vi "RT Loop - Log Data.vi"(8 "error in (no error)":errorcluster, 9 "Acceleration RT FIFO In":T1, 11 "Message Queue":refnum<queue>) -> ()   [LabVIEW 2017]
doc: "Receive triggered data from Analyze Acceleration Loop and log the data to disk."
uses:
  C:/Users/me1hlx/Desktop/Embedded Control and Monitoring/Exercises/Sample Project/support/Message Queue/Message Cluster.ctl
  C:/Users/me1hlx/Desktop/Embedded Control and Monitoring/Exercises/Sample Project/controls/Acceleration RT FIFO Reference.ctl
  C:/Users/me1hlx/Desktop/Embedded Control and Monitoring/Exercises/Sample Project/Globals/Global - All RT Loop Stop.vi
  C:/Users/me1hlx/Desktop/Embedded Control and Monitoring/Exercises/Sample Project/Globals/Global - Configuration Options.vi
  C:/Users/me1hlx/Desktop/Embedded Control and Monitoring/Exercises/Sample Project/support/Logging/Logging.lvlib
  C:/Users/me1hlx/Desktop/Embedded Control and Monitoring/Exercises/Sample Project/support/Message Queue/Message Queue.lvlib
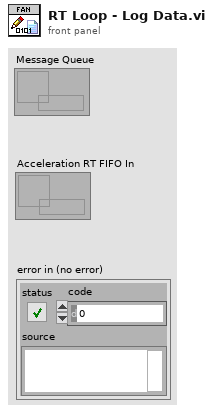
[diagram p1: front panel]
types:
  T1 = typedef "Acceleration RT FIFO Reference.ctl" = refnum<k33>
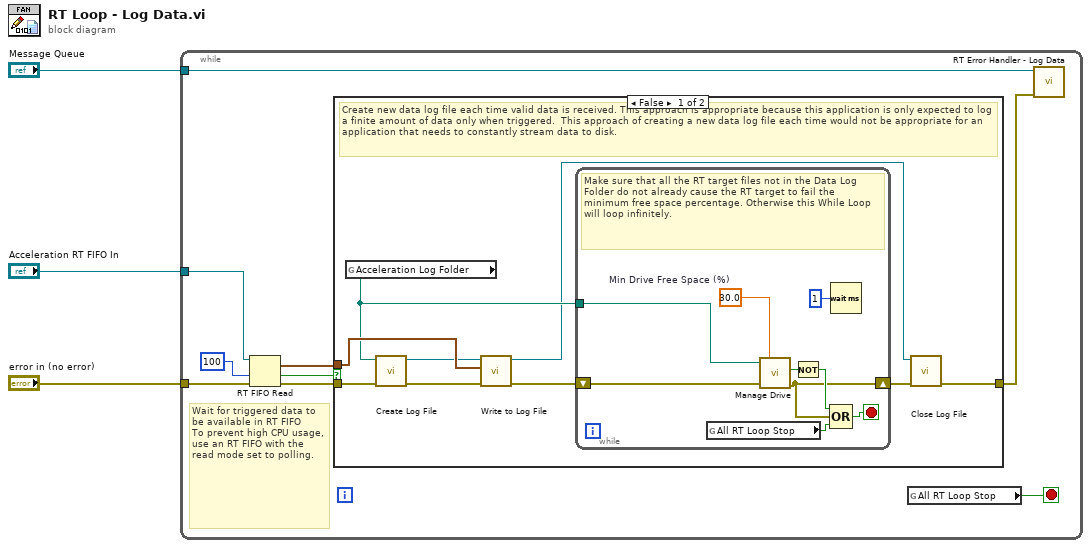
[diagram p0: block diagram]
diagram:
  n1 = while {
    tunnel: "Acceleration RT FIFO In" -> [w10]
    tunnel: "Message Queue" -> [w5]
    tunnel: "error in (no error)" -> [w12]
    stop <- w6 stop-if-true
    # "Wait for triggered data to be available in RT FIFO\nTo prevent high CPU usage, use an RT FIFO with the read mode set to polling."
    n2 = RT FIFO Read(0:w10, 2:100 ("ms timeout (0)"), 3:w12) -> (9:w7:waveform(dbl)[], 10:w8:bool, 11:w11:errorcluster)  [unwired: 1 in, 2 out]
    n3 = case shown="False" w8 {
      tunnel: w7 -> [w21 _]
      tunnel: w11 -> [w15 w31]
      tunnel: [w18 w31] -> w4
      frame False {
        # "Create new data log file each time valid data is received. This approach is appropriate because this application is only expected to log a finite amount of data only when triggered.  This approach of creating a new data log file each time would not be appropriate for an application that needs to constantly stream data to disk."
        n4 = global read "Global - Configuration Options.vi" "Acceleration Log Folder"() -> (w16:path)
        n5 = call "Create Log File.vi"("error in (no error)"=w15, "Acceleration Exceeded Log Folder"=w16) -> ("error out"=w17:errorcluster, "Log File out"=w14:refnum<k34>)  [unwired: 8 in]
        n6 = call "Write to Log File.vi"("error in (no error)"=w17, "Array of Waveforms"=w21, "Log File in"=w14) -> ("error out"=w20:errorcluster, "Log File out"=w13:refnum<k34>)  [unwired: 7 in]
        n7 = while {
          shift-right: [w25] -> w19
          shift-left: w20 -> [w26]
          tunnel: w16 -> [w23]
          stop <- w30 stop-if-true
          w24 = 30.0  # Min Drive Free Space (%)
          # "Make sure that all the RT target files not in the Data Log Folder do not already cause the RT target to fail the minimum free space percentage. Otherwise this While Loop will loop infinitely."
          n8 = global read "Global - All RT Loop Stop.vi" "All RT Loop Stop"() -> (w27:bool)
          n9 = call "Manage Drive.vi"("Min Drive Free Space (%)"=w24, "error in"=w26, "Data Folder"=w23) -> ("error out"=w25:errorcluster, "Drive Space Below Limit"=w22:bool)  [unwired: 7 in]
          n10 = Not(x=w22) -> (.not. x?=w29:bool)
          n11 = Compound Arithmetic op=OR(w29, w25, w27) -> (w30:bool)
          n12 = Wait (ms)(milliseconds to wait=u32 1) -> ()  [unwired: 1 out]
        }
        n13 = call "Close Log File.vi"("error in (no error)"=w19, "tdms file"=w13) -> ("error out"=w18:errorcluster)  [unwired: 9 in]
      }
      frame True {
        # "Timed out - No data"
      }
    }
    n14 = global read "Global - All RT Loop Stop.vi" "All RT Loop Stop"() -> (w6:bool)
    n15 = call "RT Error Handler - Log Data.vi"("error in (no error)"=w4, "Message Queue"=w5) -> ()  [unwired: 9 in, 1 out]
  }
